vi "Pause (YJ 20190221).vi"() -> ()   [LabVIEW 2017]
panel:
  in  "stop":bool
  out "Boolean":bool
  out "Paused":bool
  in  "Pause Request":bool
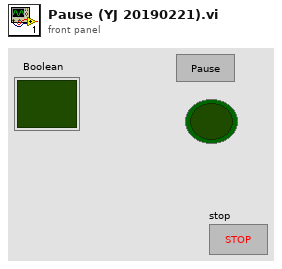
[diagram p1: front panel]
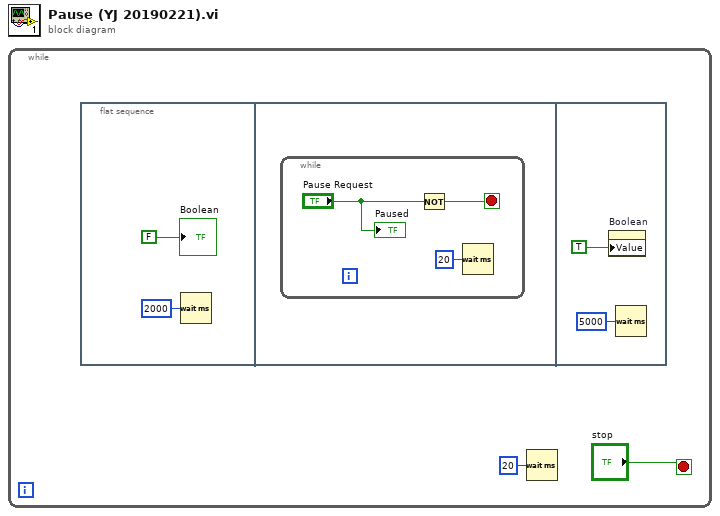
[diagram p0: block diagram]
diagram:
  n1 = while {
    stop <- "stop" stop-if-true
    n2 = flat-sequence {
      frame #0 {
        n3 = Wait (ms)(milliseconds to wait=u32 2000) -> ()  [unwired: 1 out]
        "Boolean" <- FALSE ("Boolean")
      }
      frame #1 {
        n4 = while {
          stop <- w6 stop-if-true
          n5 = Not(x="Pause Request") -> (.not. x?=w6:bool)
          n6 = Wait (ms)(milliseconds to wait=u32 20) -> ()  [unwired: 1 out]
          "Paused" <- "Pause Request"
        }
      }
      frame #2 {
        n7 = property on="Boolean" class="Bool (strict)"("Value"=TRUE ("Boolean")) -> ()  [unwired: 2 in, 2 out]
        n8 = Wait (ms)(milliseconds to wait=u32 5000) -> ()  [unwired: 1 out]
      }
    }
    n9 = Wait (ms)(milliseconds to wait=u32 20) -> ()  [unwired: 1 out]
  }
